vi "okCFrontPanelDevices Get Device & Sensors Info.vi"(8 "error in (no error)":errorcluster, 11 "okCFrontPanel Device Refnum":refnum<k24>) -> (0 "error out":errorcluster, 1 "Sensors Info":T1[](array[typedef]), 2 "Device Info":T3, 3 "okCFrontPanel Device Refnum":refnum<k24>, 4 "Device Info String":string)   [LabVIEW 2021, in "okFrontPanelC#Wrapper.lvlib"]
uses:
  okFrontPanelC#Wrapper.lvlib
  okTDeviceInfo Struct.ctl
  okEDeviceInterface.ctl
  okTFlashLayoutStruct.ctl
  okTProductID.ctl
  okEUSBSpeed.ctl
  okDeviceSensor.ctl
  okDeviceSensorType.ctl
  D:/UCLA Thinkpad Google Drive/LabVIEW 2021 SP1/builds/SwissSPAD Live Distribution/Opal Kelly/C# Wrapper/v5.0.2/libFrontPanel-csharp.dll
  v5.0.2/libFrontPanel-csharp.dll
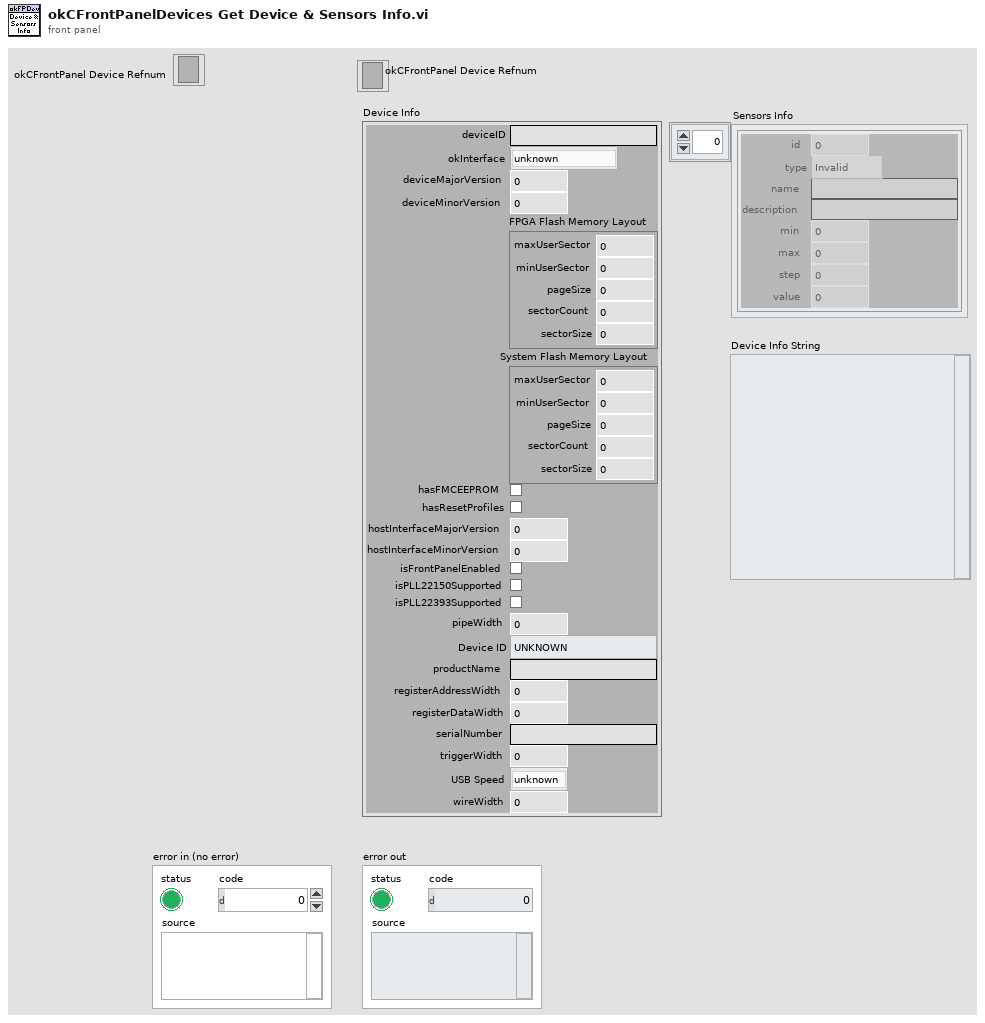
[diagram p1: front panel]
types:
  T1 = typedef "okFrontPanelC#Wrapper.lvlib/okDeviceSensor.ctl" = cluster{"id":i32, "type":T2, "name":string, "description":string, "min":dbl, "max":dbl, "step":dbl, "value":dbl}
  T2 = typedef "okFrontPanelC#Wrapper.lvlib/okDeviceSensorType.ctl" = enum16{"Invalid", "Boolean", "Integer", "Float", "Voltage", "Current", "Temperature", "Fan RPM"}
  T3 = typedef "okFrontPanelC#Wrapper.lvlib/okTDeviceInfo Struct.ctl" = cluster{"deviceID":string, "okInterface":T4, "deviceMajorVersion":i32, "deviceMinorVersion":i32, "FPGA Flash Memory Layout":T5, "System Flash Memory Layout":T5, "hasFMCEEPROM":bool, "hasResetProfiles":bool, "hostInterfaceMajorVersion":i32, "hostInterfaceMinorVersion":i32, "isFrontPanelEnabled":bool, "isPLL22150Supported":bool, "isPLL22393Supported":bool, "pipeWidth":i32, "Device ID":T6, "productName":string, "registerAddressWidth":i32, "registerDataWidth":i32, "serialNumber":string, "triggerWidth":i32, "USB Speed":T7, "wireWidth":i32}
  T4 = typedef "okFrontPanelC#Wrapper.lvlib/okEDeviceInterface.ctl" = enum16{"unknown", "USB2", "PCIe", "USB3"}
  T5 = typedef "okFrontPanelC#Wrapper.lvlib/okTFlashLayoutStruct.ctl" = cluster{"maxUserSector":u32, "minUserSector":u32, "pageSize":u32, "sectorCount":u32, "sectorSize":u32}
  T6 = typedef "okFrontPanelC#Wrapper.lvlib/okTProductID.ctl" = enum16{"UNKNOWN", "XEM3001V1", "XEM3001V2", "XEM3010", "XEM3005", "XEM3001CL", "XEM3020", "XEM3050", "XEM9002", "XEM3001RB", "XEM5010", "XEM6110LX45", "XEM6001", "XEM6010LX45", "XEM6010LX150", "XEM6110LX150", "XEM6006LX9", "XEM6006LX16", "XEM6006LX25", "XEM5010LX110", "ZEM4310", "XEM6310LX45", "XEM6310LX150", "XEM6110V2LX45", "XEM6110V2LX150", "XEM6002LX9", "XEM6310MTLX45T", "XEM6320LX130T", "XEM7350K70T", "XEM7350K160T", "XEM7350K410T", "XEM6310MTLX150T", "ZEM5305A2", "ZEM5305A7", "XEM7001A15", "XEM7001A35", "XEM7360K160T", "XEM7360K410T", "ZEM5310A4", "ZEM5310A7", "ZEM5370A5", "XEM7010A50", "XEM7010A200", "XEM7310A75", "XEM7310A200", "XEM7320A75T", "XEM7320A200T", "XEM7305", "FPXBARE"}
  T7 = typedef "okFrontPanelC#Wrapper.lvlib/okEUSBSpeed.ctl" = enum16{"unknown", "Full", "High", "Super"}
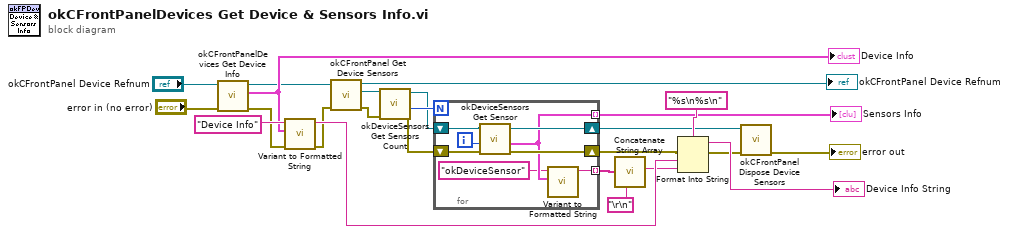
[diagram p0: block diagram]
diagram:
  n1 = call "okCFrontPanelDevices Get Device Info.vi"("error in (no error)"="error in (no error)", "okCFrontPanel Device Refnum"="okCFrontPanel Device Refnum") -> ("error out"=w17:errorcluster, "Device Info"=w16:T3, "okCFrontPanel Device Refnum"=w6:refnum<k24>)  [unwired: 7 in]
  "Device Info" <- w16
  n2 = call "Variant to Formatted String.vi"("Error In"=w17, "Variant"=w16, "Label"="Device Info") -> ("Error Out"=w22:errorcluster, "String"=w24:string)  [unwired: 7 in]
  n3 = call "okCFrontPanel Get Device Sensors.vi"("Error In"=w22, "okCFrontPanel Device Refnum"=w6) -> ("Error Out"=w9:errorcluster, "Device Sensors Refnum"=w8:refnum<k24>, "okCFrontPanel Device Refnum"=→"okCFrontPanel Device Refnum":refnum<k24>)  [unwired: 7 in]
  n4 = call "okDeviceSensors Get Sensors Count.vi"("Error In"=w9, "okDeviceSensors Refnum"=w8) -> ("Error Out"=w11:errorcluster, "Count"=w15:i32, "okDeviceSensors Refnum"=w10:refnum<k24>)  [unwired: 7 in]
  n5 = for {
    N: w15 -> [_]
    shift-right: [w28] -> w2
    shift-left: w10 -> [w32]
    shift-right: [w29] -> w23
    shift-left: w11 -> [w31]
    tunnel: [w27] -> w14 mode=indexing
    tunnel: [w26] -> w12 mode=indexing
    i -> [w30]
    n6 = call "okDeviceSensors Get Sensor.vi"("Error In"=w31, "index"=w30, "okDeviceSensors Refnum"=w32) -> ("Error Out"=w29:errorcluster, "okDeviceSensor"=w27:T1, "okDeviceSensors Refnum"=w28:refnum<k24>)  [unwired: 6 in]
    n7 = call "Variant to Formatted String.vi"("Variant"=w27, "Label"="okDeviceSensor") -> ("String"=w26:string)  [unwired: 8 in, 1 out]
  }
  "Sensors Info" <- w14
  n8 = call "Concatenate String Array.vi"("Separator (TAB)"="\r\n", "String Array"=w12) -> ("Formatted String"=w20:string)  [unwired: 9 in]
  n9 = Format Into String(format string="%s\n%s\n", error in=w23, w24, w20) -> (resulting string=→"Device Info String":string, error out=w3:errorcluster)  [unwired: 1 in]
  n10 = call "okCFrontPanel Dispose Device Sensors.vi"("Error In"=w3, "DeviceSensors Refnum"=w2) -> ("Error Out"=→"error out":errorcluster)  [unwired: 9 in]
